vi "Set Scaling.vi"(8 "error in (no error)":errorcluster, 10 "Scaling":cluster{"K":dbl, "N":dbl}[](array[cluster]), 11 "ArduinoAIReal":refnum<class "Arduino.lvclass">) -> (0 "error out":errorcluster, 3 "ArduinoAIReal":refnum<class "Arduino.lvclass">)   [LabVIEW 2020]
uses:
  Arduino.lvclass
  C:/Users/crtom/Documents/ball-beam-project.git/LabVIEW/BallBeam/ArduinoAI/ArduinoAI.lvclass
  C:/Users/crtom/Documents/ball-beam-project.git/LabVIEW/BallBeam/Arduino/Arduino.lvclass
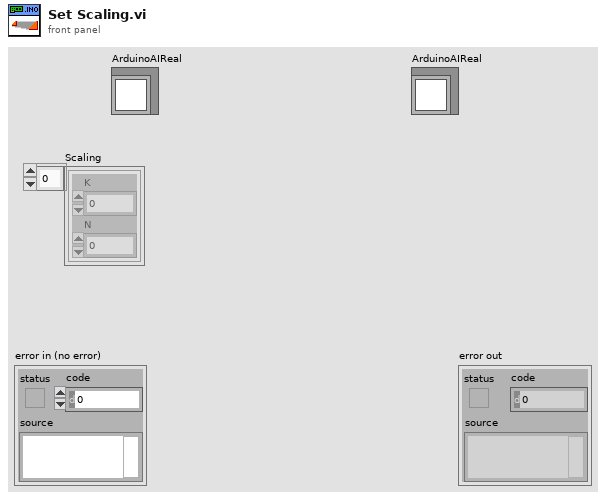
[diagram p1: front panel]
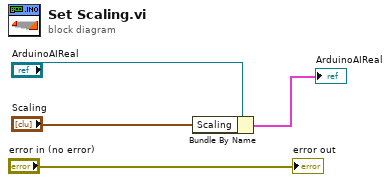
[diagram p0: block diagram]
diagram:
  n1 = Bundle By Name(cluster="ArduinoAIReal", "Scaling"="Scaling") -> (→"ArduinoAIReal":cluster{})
  "error out" <- "error in (no error)"
